vi "infusion measurables.vi"(0 "VISA resource name":refnum<visa-resource-name>, 1 "VISA wait (msec)":u32=50, 2 "Time":bool, 3 "Flow rate":bool, 4 "Volume":bool, 5 "error in (no error)":errorcluster, 8 "Mode Selector":enum16{"Withdraw", "Infuse"}(ring)=enum."Infuse") -> (14 "VISA resource name out":refnum<visa-resource-name>, 15 "Delivered volume":string, 17 "elapsed time":string, 18 "Infusion rate":string, 19 "error out":errorcluster)   [LabVIEW 2016]
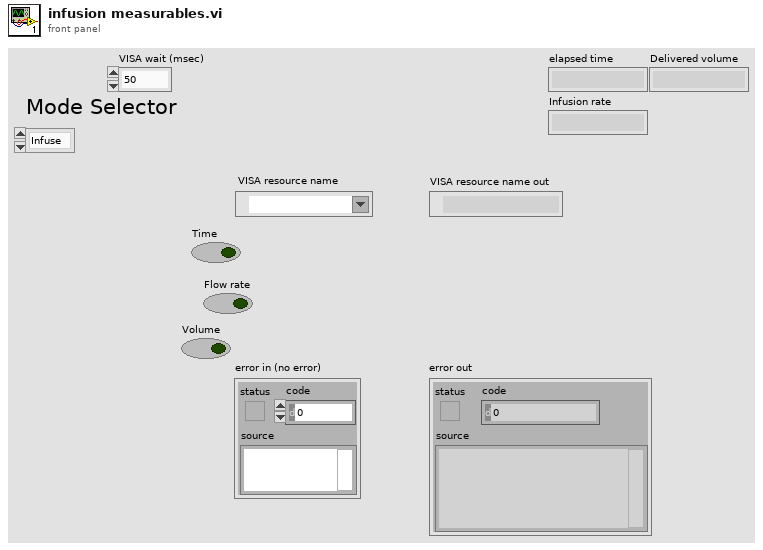
[diagram p1: front panel]
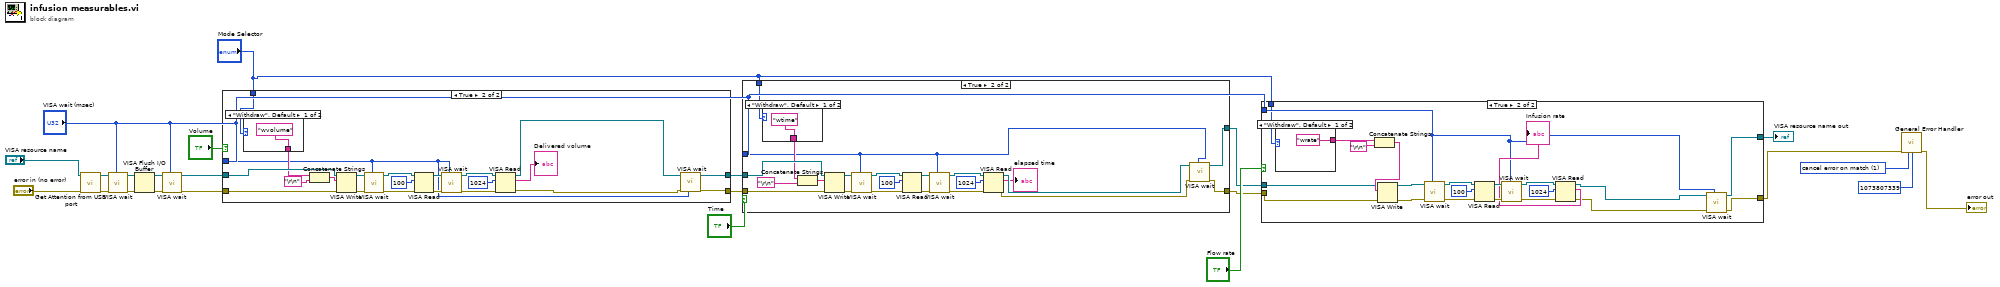
[diagram p0: block diagram]
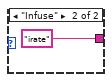
[diagram p3: hidden frame]
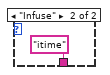
[diagram p5: hidden frame]
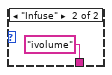
[diagram p7: hidden frame]
diagram:
  w5 = 1 items=["no exception", "cancel error on match", "set error on match"] ("[exception action] (none:0)")
  n1 = call "Get Attention from USB port.vi"("error in (no error)"="error in (no error)", "VISA resource name"="VISA resource name") -> ("error out"=w14:errorcluster, "VISA resource name out"=w15:refnum<visa-resource-name>)  [unwired: 8 in]
  n2 = call <userlib>:"VISA wait.vi"("VISA resource name"=w15, "error in (no error)"=w14, "milliseconds to wait"="VISA wait (msec)") -> ("VISA resource name out"=w13:refnum<visa-resource-name>, "error out"=w12:errorcluster)  [unwired: 6 in]
  n3 = VISA Flush I/O Buffer(VISA resource name=w13, error in (no error)=w12) -> (VISA resource name out=w19:refnum<visa-resource-name>, error out=w18:errorcluster)  [unwired: 1 in]
  n4 = call <userlib>:"VISA wait.vi"("VISA resource name"=w19, "error in (no error)"=w18, "milliseconds to wait"="VISA wait (msec)") -> ("VISA resource name out"=w17:refnum<visa-resource-name>, "error out"=w16:errorcluster)  [unwired: 6 in]
  n5 = case shown="True" "Volume" {
    tunnel: [w26 w30] -> w24
    tunnel: [w25 w31] -> w23
    tunnel: w17 -> [w26 w44]
    tunnel: w16 -> [w25 w43]
    tunnel: "VISA wait (msec)" -> [_ w29]
    tunnel: "Mode Selector" -> [_ w27]
    frame False {
    }
    frame True {
      n6 = case shown="\"Withdraw\", Default" w27 {
        tunnel: ["wvolume" ("multi-line string") "ivolume" ("multi-line string")] -> w42
        frame "Withdraw", Default {
        }
        frame "Infuse" {
        }
      }
      n7 = Concatenate Strings(w42, "\r\n") -> (w47:string)
      n8 = VISA Write(VISA resource name=w44, write buffer=w47, error in (no error)=w43) -> (VISA resource name out=w41:refnum<visa-resource-name>, error out=w40:errorcluster)  [unwired: 1 out]
      n9 = call <userlib>:"VISA wait.vi"("VISA resource name"=w41, "error in (no error)"=w40, "milliseconds to wait"=w29) -> ("VISA resource name out"=w39:refnum<visa-resource-name>, "error out"=w38:errorcluster)  [unwired: 6 in]
      n10 = VISA Read(VISA resource name=w39, byte count=u32 100, error in (no error)=w38) -> (VISA resource name out=w37:refnum<visa-resource-name>, error out=w36:errorcluster)  [unwired: 2 out]
      n11 = call <userlib>:"VISA wait.vi"("VISA resource name"=w37, "error in (no error)"=w36, "milliseconds to wait"=w29) -> ("VISA resource name out"=w35:refnum<visa-resource-name>, "error out"=w34:errorcluster)  [unwired: 6 in]
      n12 = VISA Read(VISA resource name=w35, byte count=u32 1024, error in (no error)=w34) -> (VISA resource name out=w33:refnum<visa-resource-name>, read buffer=→"Delivered volume":string, error out=w32:errorcluster)  [unwired: 1 out]
      n13 = call <userlib>:"VISA wait.vi"("VISA resource name"=w33, "error in (no error)"=w32, "milliseconds to wait"=w29) -> ("VISA resource name out"=w30:refnum<visa-resource-name>, "error out"=w31:errorcluster)  [unwired: 6 in]
    }
  }
  n14 = case shown="True" "Time" {
    tunnel: w24 -> [w52 w74]
    tunnel: w23 -> [w51 w73]
    tunnel: [w51 w58] -> w8
    tunnel: [w52 w59] -> w9
    tunnel: "VISA wait (msec)" -> [_ w57]
    tunnel: "Mode Selector" -> [_ w53]
    frame False {
    }
    frame True {
      n15 = case shown="\"Withdraw\", Default" w53 {
        tunnel: ["wtime" ("multi-line string") "itime" ("multi-line string")] -> w68
        frame "Withdraw", Default {
        }
        frame "Infuse" {
        }
      }
      n16 = Concatenate Strings(w68, "\r\n") -> (w69:string)
      n17 = VISA Write(VISA resource name=w74, write buffer=w69, error in (no error)=w73) -> (VISA resource name out=w63:refnum<visa-resource-name>, error out=w60:errorcluster)  [unwired: 1 out]
      n18 = call <userlib>:"VISA wait.vi"("VISA resource name"=w63, "error in (no error)"=w60, "milliseconds to wait"=w57) -> ("VISA resource name out"=w62:refnum<visa-resource-name>, "error out"=w61:errorcluster)  [unwired: 6 in]
      n19 = VISA Read(VISA resource name=w62, byte count=u32 100, error in (no error)=w61) -> (VISA resource name out=w67:refnum<visa-resource-name>, error out=w66:errorcluster)  [unwired: 2 out]
      n20 = call <userlib>:"VISA wait.vi"("VISA resource name"=w67, "error in (no error)"=w66, "milliseconds to wait"=w57) -> ("VISA resource name out"=w65:refnum<visa-resource-name>, "error out"=w64:errorcluster)  [unwired: 6 in]
      n21 = VISA Read(VISA resource name=w65, byte count=u32 1024, error in (no error)=w64) -> (VISA resource name out=w56:refnum<visa-resource-name>, read buffer=→"elapsed time":string, error out=w55:errorcluster)  [unwired: 1 out]
      n22 = call <userlib>:"VISA wait.vi"("VISA resource name"=w56, "error in (no error)"=w55, "milliseconds to wait"=w57) -> ("VISA resource name out"=w59:refnum<visa-resource-name>, "error out"=w58:errorcluster)  [unwired: 6 in]
    }
  }
  n23 = case shown="True" "Flow rate" {
    tunnel: w9 -> [w77 w88]
    tunnel: w8 -> [w78 w87]
    tunnel: [w78 w83] -> w3
    tunnel: [w77 w82] -> w7
    tunnel: "VISA wait (msec)" -> [_ w81]
    tunnel: "Mode Selector" -> [_ w79]
    frame False {
    }
    frame True {
      n24 = case shown="\"Withdraw\", Default" w79 {
        tunnel: ["wrate" ("string") "irate" ("string")] -> w100
        frame "Withdraw", Default {
        }
        frame "Infuse" {
        }
      }
      n25 = Concatenate Strings(w100, "\r\n") -> (w89:string)
      n26 = VISA Write(VISA resource name=w88, write buffer=w89, error in (no error)=w87) -> (VISA resource name out=w97:refnum<visa-resource-name>, error out=w96:errorcluster)  [unwired: 1 out]
      n27 = call <userlib>:"VISA wait.vi"("VISA resource name"=w97, "error in (no error)"=w96, "milliseconds to wait"=w81) -> ("VISA resource name out"=w95:refnum<visa-resource-name>, "error out"=w94:errorcluster)  [unwired: 6 in]
      n28 = VISA Read(VISA resource name=w95, byte count=u32 100, error in (no error)=w94) -> (VISA resource name out=w92:refnum<visa-resource-name>, error out=w93:errorcluster)  [unwired: 2 out]
      n29 = call <userlib>:"VISA wait.vi"("VISA resource name"=w92, "error in (no error)"=w93, "milliseconds to wait"=w81) -> ("VISA resource name out"=w91:refnum<visa-resource-name>, "error out"=w90:errorcluster)  [unwired: 6 in]
      n30 = VISA Read(VISA resource name=w91, byte count=u32 1024, error in (no error)=w90) -> (VISA resource name out=w85:refnum<visa-resource-name>, read buffer=→"Infusion rate":string, error out=w84:errorcluster)  [unwired: 1 out]
      n31 = call <userlib>:"VISA wait.vi"("VISA resource name"=w85, "error in (no error)"=w84, "milliseconds to wait"=w81) -> ("VISA resource name out"=w82:refnum<visa-resource-name>, "error out"=w83:errorcluster)  [unwired: 6 in]
    }
  }
  "VISA resource name out" <- w7
  n32 = call <vilib>:"General Error Handler.vi"("error in (no error)"=w3, "[exception action] (none:0)"=w5, "[exception code]"=1073807339) -> ("error out"=→"error out":errorcluster)  [unwired: 8 in, 4 out]
